vi "Version Number.vi"() -> (3 "Version Number":string)   [LabVIEW 2019]
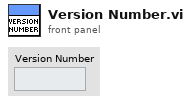
[diagram p1: front panel]
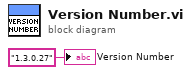
[diagram p0: block diagram]
diagram:
  "Version Number" <- "1.3.0.27" ("Version Number")
